vi "Create a Place VI Contents.vi"(6 "Variant in":variant, 7 "Shift Pressed?":bool, 8 "error in (no error)":errorcluster, 10 "QD Combo Box Ref":refnum<vi>, 11 "QD Launch VI Ref":refnum<vi>) -> (0 "error out":errorcluster, 4 "Variant out":variant)   [LabVIEW 2020, in "Create a Place VI Contents.lvlib"]
doc: "(Note: The following shortcut was originally posted by Jarrod S. on the NI Forums here. I decided to give his shortcut a more permanent home in the Quick Drop Enthusiasts group.)\n \nThis Quick Drop Keyboard Shortcut allows you to create a Place VI Contents VI (formerly called a \"Merge VI\") of your diagram selection and automatically create a user.lib palette entry for it, so that you can easily drop that selection of code in the future. Follow these steps to use this shortcut:\n \nSave the attached VI in your <LabVIEW>\\resource\\dialog\\QuickDrop\\plugins folder. No LabVIEW restart is required.\nSelect something on your diagram that you wish to make into a Place VI Contents VI.\nPress Ctrl-Space-Ctrl-Shift-G.\nSpecify a name for this Place VI Contents VI.\nCreate an icon\n \nNow you have a Place VI Contents VI that contains this diagram selection that you can use from your palettes (or Quick Drop). Note that in step (3) above, if you had pressed Ctrl-Space-Ctrl-G instead, the palettes would not be refreshed automatically, and you would have to restart LabVIEW in order to use the new Place VI Contents VI.\n \nNote: All Place VI Contents VIs that are created with this shortcut are stored in <LabVIEW Data>\\QuickDrop Templates. The actual .mnu files that provide the palette entries are stored in <LabVIEW>\\user.lib\\QuickDrop Templates Palette.mnu.\n\n\nDefault Shortcut - [G]"
uses:
  Create a Place VI Contents.lvlib
  <vilib>/Palette API/Palette Menu/Public Type Define/Palette Data.ctl
  <vilib>/Palette API/Palette Menu/Public Type Define/View Format.ctl
  <vilib>/Palette API/Palette Menu/Public Type Define/Items.ctl
  <vilib>/Palette API/Palette Menu/Public Type Define/Item.ctl
  <vilib>/Palette API/Palette Menu/Public Type Define/Help Info.ctl
  <vilib>/Palette API/Palette Menu/Public Type Define/Synchronize Info.ctl
  <vilib>/Palette API/Palette Menu/Public Type Define/Palette type.ctl
  <vilib>/Palette API/Palette Menu/Palette Menu.lvlib
panel:
  # "Do not change the connector pane of this VI."
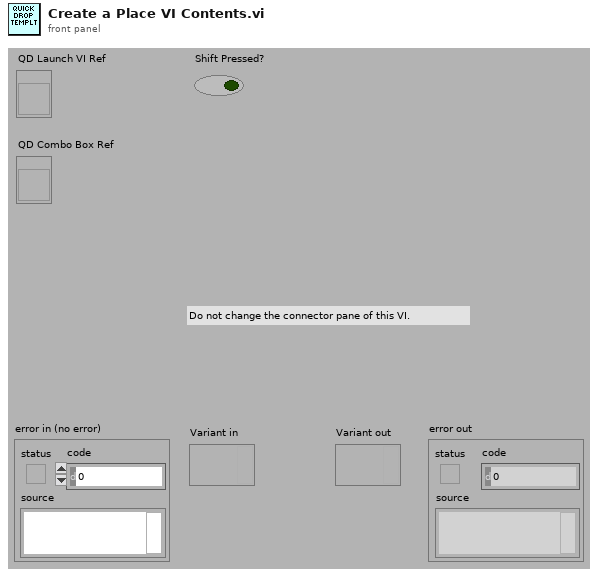
[diagram p1: front panel]
types:
  T1 = typedef "Palette Menu.lvlib/Item.ctl" = cluster{"item path":path, "library path":path, "use default lvlib palette":bool, "short name":string, "place VI contents":bool, "hide synchronized item":bool, "reserve spot for synch item":bool, "configure when placing VI contents":bool}
  T2 = typedef "Palette Menu.lvlib/Palette Data.ctl" = cluster{"display name":string, "view format":T3, "palette width":i16, "items":T4, "256 color icon":picture, "B&W color icon":picture, "help information":T5, "palette description":string, "synchronize information":T6}
  T3 = typedef "Palette Menu.lvlib/View Format.ctl" = u16
  T4 = typedef "Palette Menu.lvlib/Items.ctl" = T1[]
  T5 = typedef "Palette Menu.lvlib/Help Info.ctl" = cluster{"help tag":string, "help file path ":path}
  T6 = typedef "Palette Menu.lvlib/Synchronize Info.ctl" = cluster{"synchronize with directory":bool, "synchronize directory path":path}
  T7 = typedef "imagedata.ctl" = cluster{"image type":i32, "image depth":i32, "image":u8[], "mask":u8[], "colors":u32[], "Rectangle":cluster{"left":i16, "top":i16, "right":i16, "bottom":i16}}
  T8 = typedef "Palette Menu.lvlib/Palette type.ctl" = i32
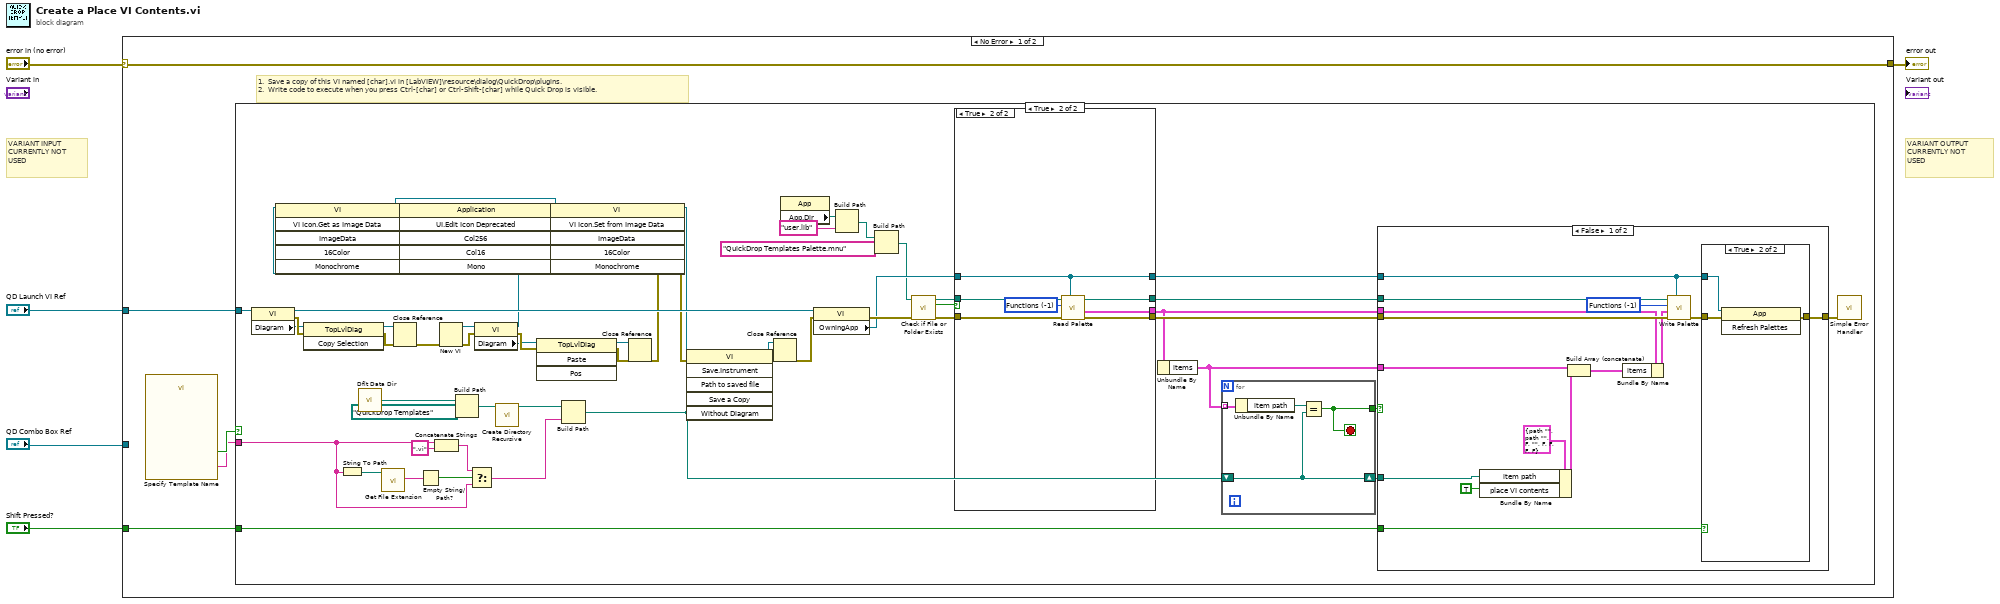
[diagram p0: block diagram]
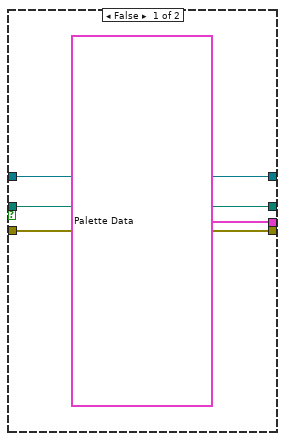
[diagram p5: hidden frame]
diagram:
  # "VARIANT INPUT\nCURRENTLY NOT\nUSED"
  # "VARIANT OUTPUT\nCURRENTLY NOT\nUSED"
  n1 = case shown="No Error" "error in (no error)" {
    selector: "error in (no error)" -> [w10 w104]
    tunnel: [w10 w104] -> w4
    tunnel: "QD Launch VI Ref" -> [w9 _]
    tunnel: "Shift Pressed?" -> [w6 _]
    tunnel: "QD Combo Box Ref" -> [_ _]
    frame No Error {
      # "1.  Save a copy of this VI named [char].vi in [LabVIEW]\\resource\\dialog\\QuickDrop\\plugins.\n2.  Write code to execute when you press Ctrl-[char] or Ctrl-Shift-[char] while Quick Drop is visible."
      n2 = call "Specify Template Name"() -> ("Template Name"=w7:string, "OK"=w8:bool)  [unwired: 17 in, 1 out]
      n3 = case shown="True" w8 {
        tunnel: w9 -> [_ w65]
        tunnel: w7 -> [_ w34]
        tunnel: w6 -> [_ w30]
        frame False {
        }
        frame True {
          n4 = property class="VI"(reference=w65) -> (reference out=w59:refnum<vi>, error out=w66:errorcluster, "Diagram"=w64:refnum<vi>)  [unwired: 1 in]
          n5 = invoke class="TopLvlDiag" method="Copy Selection"(reference=w64, error in=w66) -> (reference out=w45:refnum<vi>, error out=w44:errorcluster)  [unwired: 1 in, 1 out]
          n6 = String To Path(string=w34) -> (path=w39:path)
          n7 = call <vilib>:"Dflt Data Dir.vi"() -> ("App:Default Data Directory"=w25:path)
          n8 = call <vilib>:"Get File Extension.vi"("file"=w39) -> ("lowercase file extension"=w38:string)  [unwired: 6 in, 4 out]
          n9 = Close Reference(reference=w45, error in (no error)=w44) -> (error out=w43:errorcluster)
          n10 = Empty String/Path?(string/path=w38) -> (empty?=w37:bool)
          n11 = Concatenate Strings(w34, ".vi" ("string")) -> (w36:string)
          n12 = New VI(8:w43) -> (0:w62:errorcluster, 3:w63:refnum<vi>)  [unwired: 6 in]
          n13 = Build Path(base path=w25, name or relative path=path "QuickDrop Templates" ("App:Default Data Directory")) -> (appended path=w27:path)
          n14 = Select(t=w36, s=w37, f=w34) -> (s? t:f=w33:string)
          n15 = property class="VI"(reference=w63, error in=w62) -> (reference out=w13:refnum<vi>, error out=w68:errorcluster, "Diagram"=w61:refnum<vi>)
          n16 = call <vilib>:"Create Directory Recursive.vi"("directory"=w27) -> ("directory copy"=w24:path)  [unwired: 4 in, 2 out]
          n17 = invoke class="TopLvlDiag" method="Paste"(reference=w61, error in=w68) -> (reference out=w42:refnum<vi>, error out=w41:errorcluster)  [unwired: 2 in, 2 out]
          n18 = Build Path(base path=w24, name or relative path=w33) -> (appended path=w50:path)
          n19 = Close Reference(reference=w42, error in (no error)=w41) -> (error out=w14:errorcluster)
          n20 = invoke class="VI" method="VI Icon.Get as Image Data"(reference=w13, error in=w14) -> (reference out=w15:refnum<vi>, error out=w19:errorcluster, "ImageData"=w21:T7, "Monochrome"=w20:T7)  [unwired: 4 in, 2 out]
          n21 = invoke class="Application" method="UI.Edit Icon Deprecated"(error in=w19, "Col256"=w21, "Mono"=w20) -> (error out=w18:errorcluster, "Col256"=w17:T7, "Mono"=w16:T7)  [unwired: 3 in, 3 out]
          n22 = invoke class="VI" method="VI Icon.Set from Image Data"(reference=w15, error in=w18, "ImageData"=w17, "Monochrome"=w16) -> (reference out=w11:refnum<vi>, error out=w12:errorcluster)  [unwired: 2 in, 4 out]
          n23 = invoke class="VI" method="Save.Instrument"(reference=w11, error in=w12, "Path to saved file"=w50) -> (reference out=w40:refnum<vi>, error out=w60:errorcluster)  [unwired: 3 in, 4 out]
          n24 = Close Reference(reference=w40, error in (no error)=w60) -> (error out=w58:errorcluster)
          n25 = property class="App"() -> ("App.Dir"=w29:path)  [unwired: 2 in, 2 out]
          n26 = property class="VI"(reference=w59, error in=w58) -> (error out=w67:errorcluster, "OwningApp"=w57:refnum<vi>)  [unwired: 1 out]
          n27 = Build Path(base path=w29, name or relative path="user.lib") -> (appended path=w23:path)
          n28 = Build Path(base path=w23, name or relative path="QuickDrop Templates Palette.mnu") -> (appended path=w31:path)
          n29 = call <vilib>:"Check if File or Folder Exists.vi"("error in (no error)"=w67, "path"=w31) -> ("error out"=w54:errorcluster, "file or folder exists?"=w56:bool, "dup path"=w55:path)  [unwired: 7 in]
          n30 = case shown="True" w56 {
            tunnel: w57 -> [w93 w97]
            tunnel: w54 -> [w95 w103]
            tunnel: w55 -> [w96 w102]
            tunnel: [w96 w100] -> w52
            tunnel: [T2 {"display name"="QuickDrop Templates", "view format"=0, "palette width"=4, "items"=[], "256 color icon"=bytes[3232], "B&W color icon"=bytes[0], "help information"={"help tag"="", "help file path "=path ""}, "palette description"="", "synchronize information"={"synchronize with directory"=FALSE, "synchronize directory path"=path ""}} ("palette data") w99] -> w51
            tunnel: [w95 w98] -> w53
            tunnel: [w93 w97] -> w46
            frame False {
            }
            frame True {
              w101 = T8 -1 items=["Functions"=-1, "Controls"=-2] ("palette type")
              n31 = call <vilib>:"Read Palette.vi"("application reference"=w97, "error in (no error)"=w103, "palette type"=w101, "palette path"=w102) -> ("error out"=w98:errorcluster, "palette data"=w99:T2, "duplicate palette path"=w100:path)  [unwired: 5 in]
            }
          }
          n32 = Unbundle By Name(w51) -> ("items"=w48:T4)
          n33 = for {
            tunnel: w48 -> [w92] mode=indexing
            tunnel: [w90] -> w49
            shift-right: [w89] -> w47
            shift-left: w50 -> [w89]
            stop <- w90 stop-if-true
            n34 = Unbundle By Name(w92) -> ("item path"=w91:path)
            n35 = Equal?(x=w91, y=w89) -> (x = y?=w90:bool)
          }
          n36 = case shown="False" w49 {
            tunnel: w53 -> [w82 w88]
            tunnel: w52 -> [w81 _]
            tunnel: w51 -> [w79 _]
            tunnel: w48 -> [w78 _]
            tunnel: w47 -> [w75 _]
            tunnel: w46 -> [w69 _]
            tunnel: w30 -> [w71 _]
            tunnel: [w70 w88] -> w22
            frame False {
              w83 = T8 -1 items=["Functions"=-1, "Controls"=-2] ("palette type")
              n37 = Bundle By Name(cluster=T1 {"item path"=path "", "library path"=path "", "use default lvlib palette"=FALSE, "short name"="", "place VI contents"=FALSE, "hide synchronized item"=FALSE, "reserve spot for synch item"=FALSE, "configure when placing VI contents"=FALSE} ("Items"), "item path"=w75, "place VI contents"=TRUE) -> (w76:T1)
              n38 = Build Array (concatenate)(w78, w76) -> (w73:T4)
              n39 = Bundle By Name(cluster=w79, "items"=w73) -> (w80:T2)
              n40 = call <vilib>:"Write Palette.vi"("application reference"=w69, "error in (no error)"=w82, "palette data"=w80, "palette type"=w83, "palette path"=w81) -> ("error out"=w72:errorcluster)  [unwired: 6 in]
              n41 = case shown="True" w71 {
                tunnel: w69 -> [_ w87]
                tunnel: w72 -> [w84 w86]
                tunnel: [w84 w85] -> w70
                frame False {
                }
                frame True {
                  n42 = invoke class="App" method="Refresh Palettes"(reference=w87, error in=w86) -> (error out=w85:errorcluster)  [unwired: 1 in, 2 out]
                }
              }
            }
            frame True {
              # "Item already exists in palette."
            }
          }
          n43 = call <vilib>:"Simple Error Handler.vi"("error in (no error)"=w22) -> ()  [unwired: 4 in, 5 out]
        }
      }
    }
    frame Error {
    }
  }
  "error out" <- w4
